vi "Extract Number of Image in Set.vi"(8 "Error In":errorcluster, 11 "Image Name":string="IMG_0020_1.tif") -> (0 "Error Out":errorcluster, 3 "Number of pics taken":i32)   [LabVIEW 2014]
panel:
  out "after substring":string
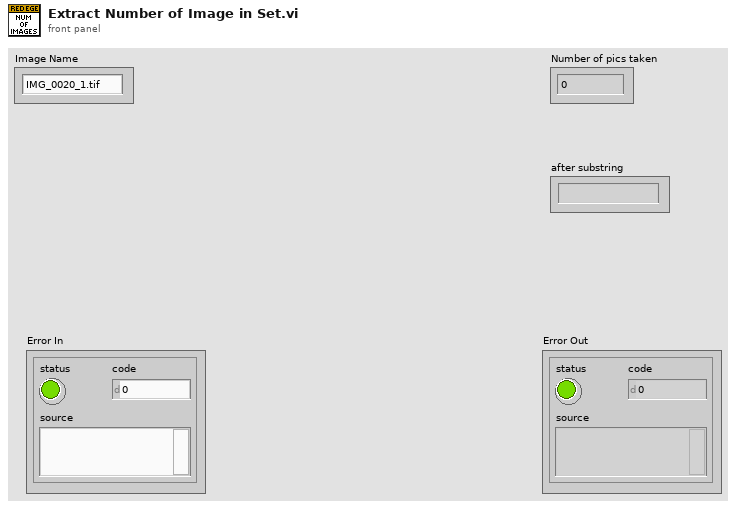
[diagram p1: front panel]
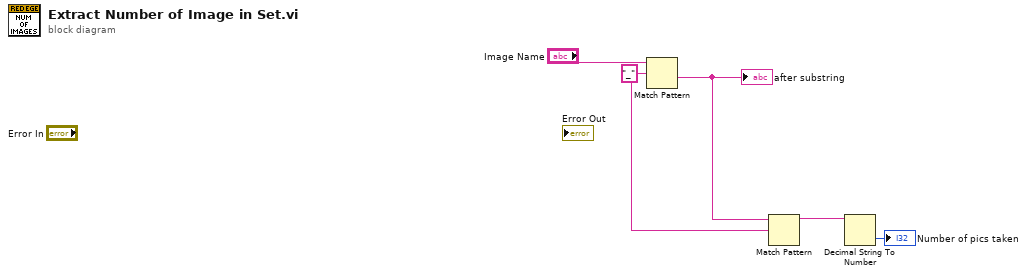
[diagram p0: block diagram]
diagram:
  w3 = "_" ("regular expression")
  n1 = Match Pattern(string="Image Name", regular expression=w3) -> (after substring=w4:string)  [unwired: 1 in, 3 out]
  "after substring" <- w4
  n2 = Match Pattern(string=w4, regular expression=w3) -> (before substring=w2:string)  [unwired: 1 in, 3 out]
  n3 = Decimal String To Number(string=w2) -> (number=→"Number of pics taken":i32)  [unwired: 2 in, 1 out]
